vi "PusherServo Close.vi"(8 "error in (no error)":errorcluster, 11 "ServoDeviceRef Out":T1) -> (0 "error out":errorcluster)   [LabVIEW 2023, in "Feeder_ACT.lvlib"]
uses:
  Feeder_ACT.lvlib
  <vilib>/Rock Robotics/WPI/PWM/Servo/WPI_ServoDeviceRef.ctl
  <vilib>/Rock Robotics/SystemInterfaces/DIO/FPGA_DIOPWMChannel.ctl
  <vilib>/Rock Robotics/WPI/PWM/WPI_PWMDeadband.ctl
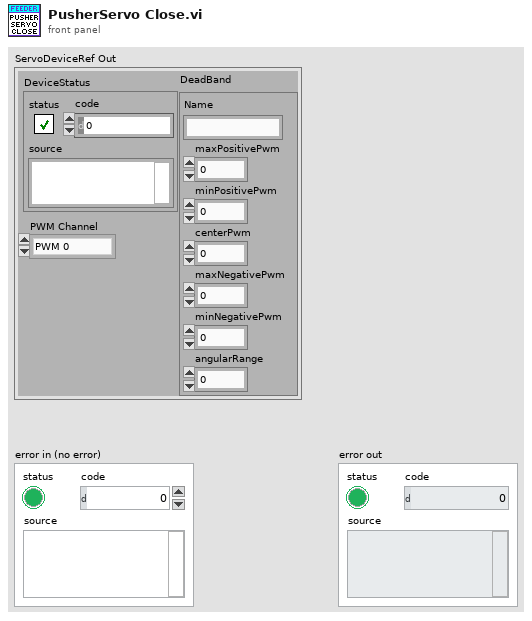
[diagram p1: front panel]
types:
  T1 = typedef "WPI_ServoDeviceRef.ctl" = cluster{"DeviceStatus":errorcluster, "PWM Channel":T2, "DeadBand":T3}
  T2 = typedef "FPGA_DIOPWMChannel.ctl" = enum8{"PWM 0", "PWM 1", "PWM 2", "PWM 3", "PWM 4", "PWM 5", "PWM 6", "PWM 7", "PWM 8", "PWM 9", "PWM MXP 0", "PWM MXP 1", "PWM MXP 2", "PWM MXP 3", "PWM MXP 4", "PWM MXP 5", "PWM MXP 6", "PWM MXP 7", "PWM MXP 8", "PWM MXP 9", "Invalid"}
  T3 = typedef "WPI_PWMDeadband.ctl" = cluster{"Name":string, "maxPositivePwm":i32, "minPositivePwm":i32, "centerPwm":i32, "maxNegativePwm":i32, "minNegativePwm":i32, "angularRange":u16}
  T4 = typedef "WPI_PWMDeviceRef.ctl" = cluster{"DeviceStatus":errorcluster, "PWM Channel":T2}
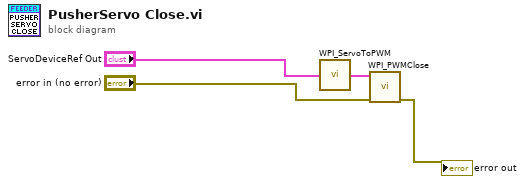
[diagram p0: block diagram]
diagram:
  n1 = call <vilib>:"WPI_ServoToPWM.vi"("ServoDeviceRef"="ServoDeviceRef Out") -> ("PWMDeviceRef"=w1:T4)
  n2 = call <vilib>:"WPI_PWMClose.vi"("error in (no error)"="error in (no error)", "PWMDeviceRef"=w1) -> ("error out"=→"error out":errorcluster)  [unwired: 9 out]
